vi "Grey Scale Color Table.vi"() -> ()   [LabVIEW 2022 SP3]
panel:
  out "Intensity Graph":dbl[][](graph)
  in  "grayscale  table":u32[](array[numeric])=[0, 16777215, 16711421, 16645628, 16514042, 16448249, 16316663, 16250870, 16119284, 16053491, 15921905, 15856112, 15724526, 15658733, 15527147, 15461354, 15395561, 15263975, 15198182, 15066596, 15000803, 14935010, 14869217, 14803424, 14737631, 14671838, 14606045, 14606045, 14540252, 14474459, 14408666, 14342873, 14277080, 14211287, 14145494, 14079701, 14013908, 13948115, 13882322, 13816529, 13750736, 13684943, 13619150, 13553357, 13487564, 13421771, 13355978, 13290185, 13224392, 13158599, 13092806, 13027013, 12961220, 12895427, 12829634, 12763841, 12698048, 12632255, 12566462, 12566462, 12500669, 12434876, 12369083, 12303290, 12237497, 12171704, 12105911, 12040118, 11974325, 11908532, 11842739, 11776946, 11711153, 11645360, 11579567, 11513774, 11447981, 11382188, 11316395, 11250602, 11184809, 11119016, 11053223, 10987430, 10921637, 10855844, 10790051, 10724258, 10658465, 10592672, 10526879, 10461086, 10461086, 10395293, 10329500, 10263707, 10197914, 10132121, 10066328, 10000535, 9934742, 9868949, 9803156, 9737363, 9671570, 9605777, 9539984, 9474191, 9408398, 9342605, 9276812, 9211019, 9145226, 9079433, 9013640, 8947847, 8882054, 8816261, 8750468, 8684675, 8618882, 8553089, 8487296, 8421503, 8355710, 8355710, 8289917, 8224124, 8158331, 8092538, 8026745, 7960952, 7895159, 7829366, 7763573, 7697780, 7631987, 7566194, 7500401, 7434608, 7368815, 7303022, 7237229, 7171436, 7105643, 7039850, 6974057, 6908264, 6842471, 6776678, 6710885, 6645092, 6579299, 6513506, 6447713, 6381920, 6316127, 6316127, 6250334, 6184541, 6118748, 6052955, 5987162, 5921369, 5855576, 5789783, 5723990, 5658197, 5592404, 5526611, 5460818, 5395025, 5329232, 5263439, 5197646, 5131853, 5066060, 5000267, 4934474, 4868681, 4802888, 4737095, 4671302, 4605509, 4539716, 4473923, 4408130, 4342337, 4276544, 4210751, 4210751, 4144958, 4079165, 4013372, 3947579, 3881786, 3815993, 3750200, 3684407, 3618614, 3552821, 3487028, 3421235, 3355442, 3289649, 3223856, 3158063, 3092270, 3026477, 2960684, 2894891, 2829098, 2763305, 2697512, 2631719, 2565926, 2500133, 2434340, 2368547, 2302754, 2236961, 2171168, 2105375, 2105375, 2039582, 1973789, 1907996, 1842203, 1776410, 1710617, 1644824, 1579031, 1513238, 1447445, 1381652, 1315859, 1250066, 1184273, 1118480, 1052687, 986894, 921101, 855308, 789515, 723722, 657929, 592136, 526343, 460550, 394757, 328964, 263171, 197378, 131585, 65792, 16777215]
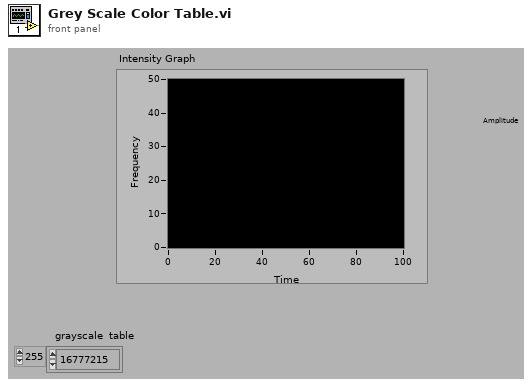
[diagram p1: front panel]
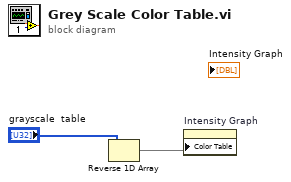
[diagram p0: block diagram]
diagram:
  n1 = Reverse 1D Array(array="grayscale  table") -> (reversed array=w1:u32[])
  n2 = property on="Intensity Graph" class="IntGraph (strict)"("Color Table"=w1) -> ()  [unwired: 2 in, 2 out]
